vi "OMEGA_Temp.vi"() -> ()   [LabVIEW 2020]
uses:
  <vilib>/Utility/error.llb/DialogType.ctl
  <vilib>/ULx/Create Channel.llb/ULx Create Channel (AI-Temperature).vi
  <vilib>/ULx/Read.llb/ULx Read (Analog 1D Wfm NChan NSamp).vi
panel:
  in  "stop":bool
  out "Tempurature Chart":waveform(dbl)[](graph)
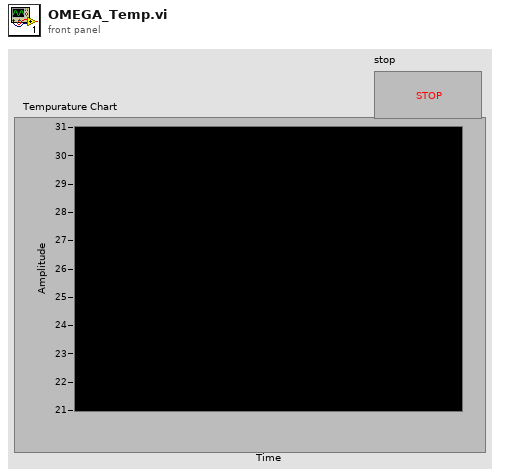
[diagram p1: front panel]
types:
  T1 = typedef "DialogType.ctl" = u16
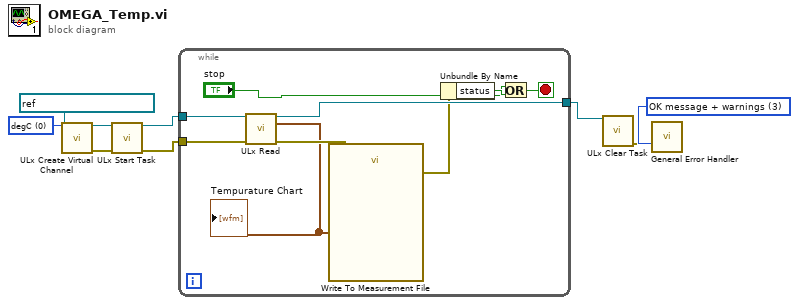
[diagram p0: block diagram]
diagram:
  w3 = 0 items=["degC", "degF", "kelvin", "raw"] ("units")
  w9 = T1 3 items=["no dialog", "OK message", "continue or stop message", "OK message + warnings", "continue/stop + warnings"] ("type of dialog (OK msg:1)")
  n1 = call-poly <vilib>:"ULx Create Virtual Channel.vi"("physical channels"=refnum<k21> "Dev1/Ti0, Dev1/Ti1", "units"=w3) -> ("task out"=w2:refnum<k24>, "error out"=w1:errorcluster)  [unwired: 12 in]
  n2 = call <vilib>:"ULx Start Task.vi"("task in"=w2, "error in"=w1) -> ("task out"=w6:refnum<k24>, "error out"=w5:errorcluster)  [unwired: 12 in]
  n3 = while {
    tunnel: w5 -> [w15]
    tunnel: w6 -> [w18]
    tunnel: [w17] -> w7
    stop <- w16 stop-if-true
    n4 = call-poly <vilib>:"ULx Read.vi"("task in"=w18, "error in"=w15) -> ("task out"=w17:refnum<k24>, "data"=w11:waveform(dbl)[], "error out"=w13:errorcluster)  [unwired: 11 in]
    "Tempurature Chart" <- w11
    n5 = call "Write To Measurement File"("Signals"=w11, "error in (no error)"=w13) -> ("error out"=w12:errorcluster)  [unwired: 15 in, 2 out]
    n6 = Unbundle By Name(w12) -> ("status"=w14:bool)
    n7 = Or(x="stop", y=w14) -> (x .or. y?=w16:bool)
  }
  n8 = call <vilib>:"ULx Clear Task.vi"("task in"=w7) -> ("error out"=w8:errorcluster)  [unwired: 14 in]
  n9 = call <vilib>:"General Error Handler.vi"("type of dialog (OK msg:1)"=w9, "error in (no error)"=w8) -> ()  [unwired: 9 in, 5 out]
